vi "delete mapping by tag helper.vi"(9 "input channel?":bool, 10 "tag name":string, 11 "Mappings":T1[](array[typedef])) -> (3 "Mappings out":T1[](array[typedef]))   [LabVIEW 2013, in "engine configuration.lvclass"]
uses:
  engine configuration.lvclass
  <vilib>/NI/Tag Bus/table/mapping specification.ctl
  <vilib>/NI/Tag Bus/tag/Data Type.ctl
  <vilib>/NI/Tag Bus/table/mapping.ctl
  <vilib>/NI/Tag Bus/tag/tag descriptor.lvclass
  <vilib>/NI/Tag Bus/table/data table.lvlib
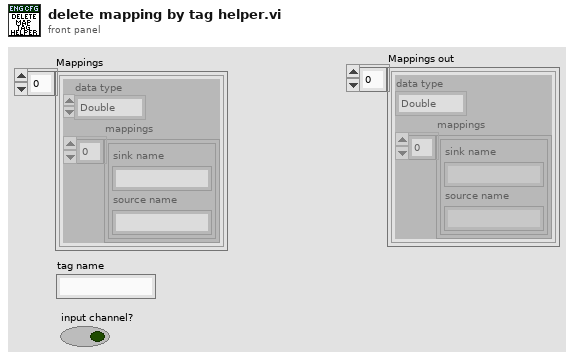
[diagram p1: front panel]
types:
  T1 = typedef "tag bus.lvlib/data table.lvlib/mapping specification.ctl" = cluster{"data type":T2, "mappings":T3[]}
  T2 = typedef "tag bus.lvlib/tag descriptor.lvclass/Data Type.ctl" = enum16{"Double", "Single", "I64", "I32", "I16", "I8", "U64", "U32", "U16", "U8", "Boolean", "String", "Array of Double", "Array of Single", "Array of I64", "Array of I32", "Array of I16", "Array of I8", "Array of U64", "Array of U32", "Array of U16", "Array of U8", "Array of Boolean", "Array of String"}
  T3 = typedef "tag bus.lvlib/data table.lvlib/mapping.ctl" = cluster{"sink name":string, "source name":string}
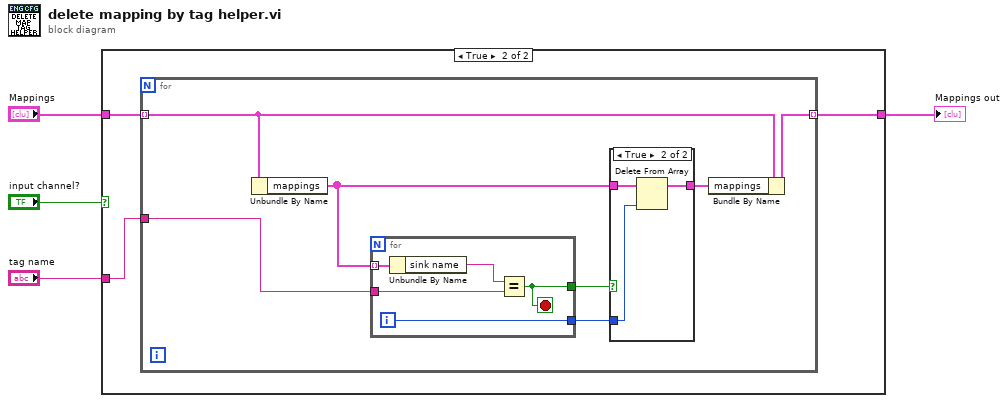
[diagram p0: block diagram]
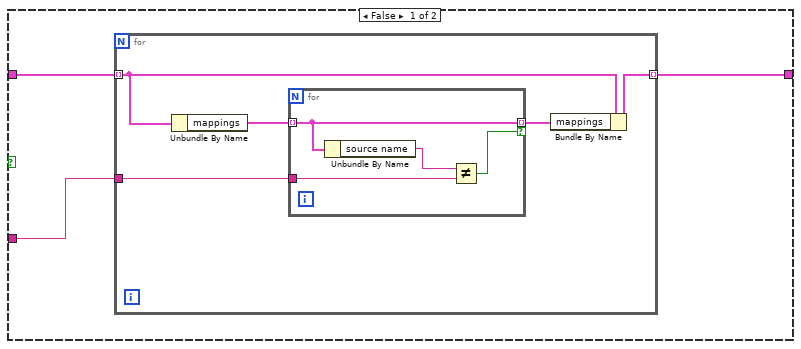
[diagram p2: hidden frame]
diagram:
  n1 = case shown="True" "input channel?" {
    tunnel: "Mappings" -> [w7 w19]
    tunnel: "tag name" -> [w6 w18]
    tunnel: [w5 w17] -> w1
    frame False {
      n2 = for {
        tunnel: w7 -> [w10] mode=indexing
        tunnel: w6 -> [w11]
        tunnel: [w8] -> w5 mode=indexing
        n3 = Unbundle By Name(w10) -> ("mappings"=w12:T3[])
        n4 = for {
          tunnel: w12 -> [w14] mode=indexing
          tunnel: w11 -> [w15]
          tunnel: [w14] -> w9 mode=indexing if=w13
          n5 = Unbundle By Name(w14) -> ("source name"=w16:string)
          n6 = Not Equal?(x=w16, y=w15) -> (x != y?=w13:bool)
        }
        n7 = Bundle By Name(cluster=w10, "mappings"=w9) -> (w8:T1)
      }
    }
    frame True {
      n8 = for {
        tunnel: w19 -> [w26] mode=indexing
        tunnel: [w25] -> w17 mode=indexing
        tunnel: w18 -> [w24]
        n9 = Unbundle By Name(w26) -> ("mappings"=w22:T3[])
        n10 = for {
          tunnel: w22 -> [w35] mode=indexing
          tunnel: w24 -> [w33]
          tunnel: [w32] -> w20
          tunnel: [w31] -> w23
          i -> [w32]
          stop <- w31 stop-if-true
          n11 = Unbundle By Name(w35) -> ("sink name"=w34:string)
          n12 = Equal?(x=w34, y=w33) -> (x = y?=w31:bool)
        }
        n13 = case shown="True" w23 {
          tunnel: w22 -> [w27 w30]
          tunnel: [w27 w29] -> w21
          tunnel: w20 -> [_ w28]
          frame False {
          }
          frame True {
            n14 = Delete From Array(array=w30, index=w28) -> (array with subset deleted=w29:T3[])  [unwired: 1 in, 1 out]
          }
        }
        n15 = Bundle By Name(cluster=w26, "mappings"=w21) -> (w25:T1)
      }
    }
  }
  "Mappings out" <- w1
